vi "DMM Mixed Meas Format Function Range.vi"(0 "DMM Handle In":refnum<k15>, 5 "Function Settings In":T1={"Range and Function"=enum."DC Voltage Auto Range", "Resolution in Digits"=5.5} {"Resolution in Digits" items=["3 1/2"=3.5, "4 1/2"=4.5, "5 1/2"=5.5, "6 1/2"=6.5, "7 1/2"=7.5]}, 11 "error in":errorcluster) -> (4 "DMM Handle Out":refnum<k15>, 6 "Function Settings Out":T4={"Range"=0.0, "Function"=enum."DC Volts", "AC Range"=0.0, "Resolution in Digits"=5.5} {"Resolution in Digits" items=["3 1/2"=3.5, "4 1/2"=4.5, "5 1/2"=5.5, "6 1/2"=6.5, "7 1/2"=7.5]}, 15 "error out":errorcluster)   [LabVIEW 2021, in "DMM_Mixed Measurement.lvlib"]
doc: "Utilizes the function settings input to select the particular function and range used for the measurement and format the output string displayed in the measurement output cluster."
uses:
  DMM_Mixed Measurement.lvlib
  <instrlib>/niDMM/nidmm.llb/niDMM Function.ctl
  <instrlib>/niDMM/nidmm.llb/niDMM Resolution in Digits.ctl
  DMM Mixed Meas Typedefs/Function Settings.ctl
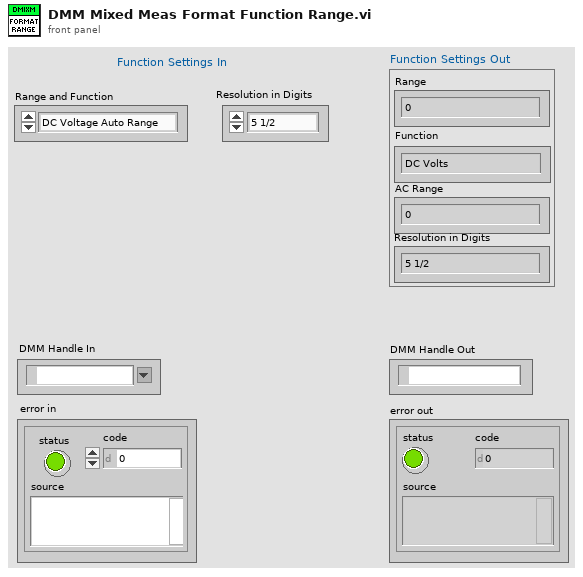
[diagram p1: front panel]
types:
  T1 = typedef "DMM_Mixed Measurement.lvlib/Function Settings.ctl" = cluster{"Range and Function":enum16{"DC Voltage Auto Range", "DC 100 mV", "DC 1 V ", "DC 10 V", "DC 100 V", "DC 300 V", " ", "AC Voltage Auto Range", "AC 50 mV", "AC 200 mV", "AC 500 mV", "AC 2 V", "AC 5 V", "AC 20 V", "AC 50 V", "AC 300 V", "  ", "DC Current Auto Range", "DC 1 uA", "DC 10 uA", "DC 100 uA", "DC 1 mA", "DC 10 mA", "DC 20 mA", "DC 100 mA", "DC 200 mA", "DC 1 A", "DC 3 A", "   ", "AC Current Auto Range", "AC 100 uA", "AC 1 mA", "AC 10 mA", "AC 100 mA", "AC 500 mA", "AC 1 A", "AC 3 A", "    ", "Resistance Auto Range", "Res 100 Ohm", "Res 1 kOhm", "Res 10 kOhm", "Res 100 kOhm", "Res 1 MOhm", "Res 10 MOhm", "Res 100 MOhm", "Res 5 GOhm", "     ", "Frequency AC Auto Range", "Freq AC 50 mV", "Freq AC 500 mV", "Freq AC 5 V", "Freq AC 50 V", "Freq AC 300 V", "      ", "Period AC Auto Range", "Period AC 50 mV", "Period AC 500 mV", "Period AC 5 V", "Period AC 50 V", "Period AC 300 V"}, "Resolution in Digits":T2}
  T2 = typedef "niDMM Resolution in Digits.ctl" = dbl
  T3 = typedef "niDMM Function.ctl" = enum16{"DC Volts", "AC Volts", "DC Current", "AC Current", "2-wire Resistance", "4-wire Resistance", "Diode", "Frequency", "Period", "AC Volts DC Coupled", "Capacitance", "Inductance", "Temperature"}
  T4 = cluster{"Range":dbl, "Function":T3, "AC Range":dbl, "Resolution in Digits":T2}
  T5 = cluster{"Range":dbl, "Function":T3, "Freq_Period AC Range":dbl, "Resolution in Digits":T2}
  T6 = enum16{"DC Voltage Auto Range", "DC 100 mV", "DC 1 V ", "DC 10 V", "DC 100 V", "DC 300 V", " ", "AC Voltage Auto Range", "AC 50 mV", "AC 200 mV", "AC 500 mV", "AC 2 V", "AC 5 V", "AC 20 V", "AC 50 V", "AC 300 V", "  ", "DC Current Auto Range", "DC 1 uA", "DC 10 uA", "DC 100 uA", "DC 1 mA", "DC 10 mA", "DC 20 mA", "DC 100 mA", "DC 200 mA", "DC 1 A", "DC 3 A", "   ", "AC Current Auto Range", "AC 100 uA", "AC 1 mA", "AC 10 mA", "AC 100 mA", "AC 500 mA", "AC 1 A", "AC 3 A", "    ", "Resistance Auto Range", "Res 100 Ohm", "Res 1 kOhm", "Res 10 kOhm", "Res 100 kOhm", "Res 1 MOhm", "Res 10 MOhm", "Res 100 MOhm", "Res 5 GOhm", "     ", "Frequency AC Auto Range", "Freq AC 50 mV", "Freq AC 500 mV", "Freq AC 5 V", "Freq AC 50 V", "Freq AC 300 V", "      ", "Period AC Auto Range", "Period AC 50 mV", "Period AC 500 mV", "Period AC 5 V", "Period AC 50 V", "Period AC 300 V"}
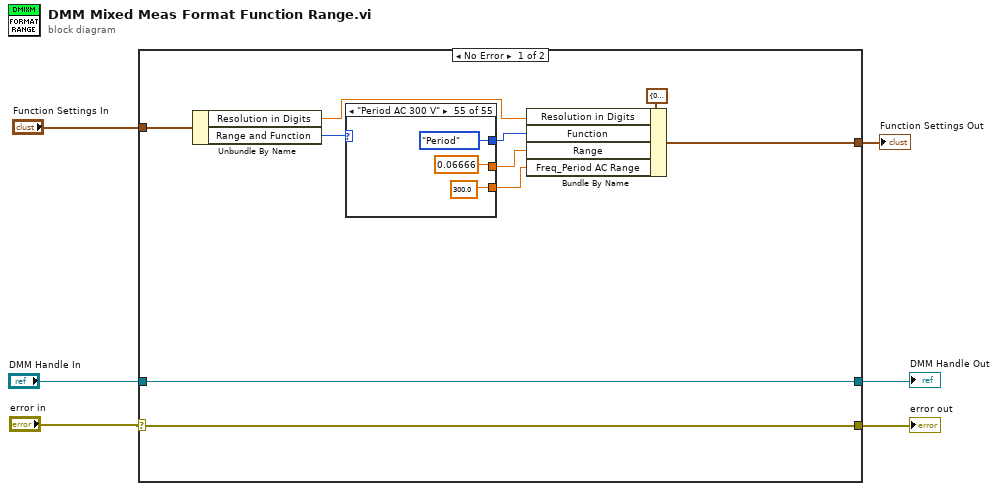
[diagram p0: block diagram]
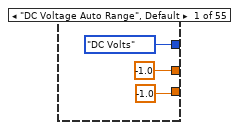
[diagram p2: hidden frame]
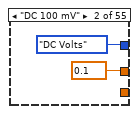
[diagram p3: hidden frame]
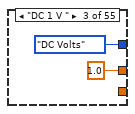
[diagram p4: hidden frame]
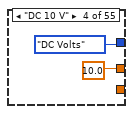
[diagram p5: hidden frame]
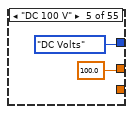
[diagram p6: hidden frame]
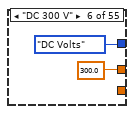
[diagram p7: hidden frame]
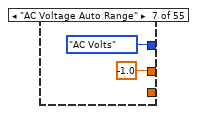
[diagram p8: hidden frame]
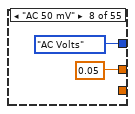
[diagram p9: hidden frame]
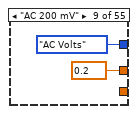
[diagram p10: hidden frame]
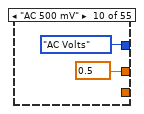
[diagram p11: hidden frame]
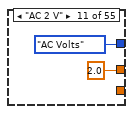
[diagram p12: hidden frame]
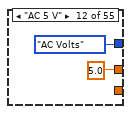
[diagram p13: hidden frame]
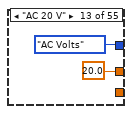
[diagram p14: hidden frame]
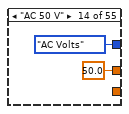
[diagram p15: hidden frame]
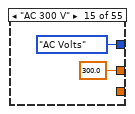
[diagram p16: hidden frame]
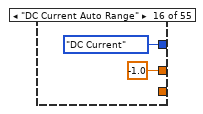
[diagram p17: hidden frame]
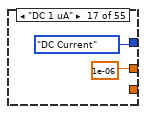
[diagram p18: hidden frame]
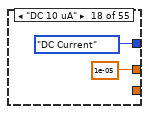
[diagram p19: hidden frame]
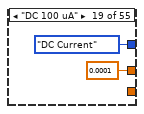
[diagram p20: hidden frame]
diagram:
  n1 = case shown="No Error" "error in" {
    selector: "error in" -> [w8 w141]
    tunnel: "Function Settings In" -> [w16 _]
    tunnel: [w9 T5 {"Range"=-1.0, "Function"=enum."DC Volts", "Freq_Period AC Range"=-1.0, "Resolution in Digits"=5.5} ("Function Settings")] -> w2
    tunnel: [w8 w141] -> w5
    tunnel: [w7 w142] -> w3
    tunnel: "DMM Handle In" -> [w7 w142]
    frame No Error {
      n2 = Unbundle By Name(w16) -> ("Resolution in Digits"=w14:T2, "Range and Function"=w15:T6)
      n3 = case shown="\"Period AC 300 V\"" w15 {
        tunnel: [niDMM_Function."DC Volts" ("Function") niDMM_Function."DC Volts" ("Function") niDMM_Function."DC Volts" ("Function") niDMM_Function."DC Volts" ("Function") niDMM_Function."DC Volts" ("Function") niDMM_Function."DC Volts" ("Function") niDMM_Function."AC Volts" ("Function") niDMM_Function."AC Volts" ("Function") niDMM_Function."AC Volts" ("Function") niDMM_Function."AC Volts" ("Function") niDMM_Function."AC Volts" ("Function") niDMM_Function."AC Volts" ("Function") niDMM_Function."AC Volts" ("Function") niDMM_Function."AC Volts" ("Function") niDMM_Function."AC Volts" ("Function") niDMM_Function."DC Current" ("Function") niDMM_Function."DC Current" ("Function") niDMM_Function."DC Current" ("Function") niDMM_Function."DC Current" ("Function") niDMM_Function."DC Current" ("Function") niDMM_Function."DC Current" ("Function") niDMM_Function."DC Current" ("Function") niDMM_Function."DC Current" ("Function") niDMM_Function."DC Current" ("Function") niDMM_Function."DC Current" ("Function") niDMM_Function."DC Current" ("Function") niDMM_Function."AC Current" ("Function") niDMM_Function."AC Current" ("Function") niDMM_Function."AC Current" ("Function") niDMM_Function."AC Current" ("Function") niDMM_Function."AC Current" ("Function") niDMM_Function."AC Current" ("Function") niDMM_Function."AC Current" ("Function") niDMM_Function."AC Current" ("Function") niDMM_Function."2-wire Resistance" ("Function") niDMM_Function."2-wire Resistance" ("Function") niDMM_Function."2-wire Resistance" ("Function") niDMM_Function."2-wire Resistance" ("Function") niDMM_Function."2-wire Resistance" ("Function") niDMM_Function."2-wire Resistance" ("Function") niDMM_Function."2-wire Resistance" ("Function") niDMM_Function."2-wire Resistance" ("Function") niDMM_Function."2-wire Resistance" ("Function") niDMM_Function."Frequency" ("Function") niDMM_Function."Frequency" ("Function") niDMM_Function."Frequency" ("Function") niDMM_Function."Frequency" ("Function") niDMM_Function."Frequency" ("Function") niDMM_Function."Frequency" ("Function") niDMM_Function."Period" ("Function") niDMM_Function."Period" ("Function") niDMM_Function."Period" ("Function") niDMM_Function."Period" ("Function") niDMM_Function."Period" ("Function") niDMM_Function."Period" ("Function")] -> w10
        tunnel: [-1.0 ("Range") 0.1 ("Range") 1.0 ("Range") 10.0 ("Range") 100.0 ("Range") 300.0 ("Range") -1.0 ("Range") 0.05 ("Range") 0.2 ("Range") 0.5 ("Range") 2.0 ("Range") 5.0 ("Range") 20.0 ("Range") 50.0 ("Range") 300.0 ("Range") -1.0 ("Range") 1e-06 ("Range") 1e-05 ("Range") 0.0001 ("Range") 0.001 ("Range") 0.01 ("Range") 0.02 ("Range") 0.1 ("Range") 0.2 ("Range") 1.0 ("Range") 3.0 ("Range") -1.0 ("Range") 0.0001 ("Range") 0.001 ("Range") 0.01 ("Range") 0.1 ("Range") 0.5 ("Range") 1.0 ("Range") 3.0 ("Range") -1.0 ("Range") 100.0 ("Range") 1000.0 ("Range") 10000.0 ("Range") 100000.0 ("Range") 1000000.0 ("Range") 10000000.0 ("Range") 100000000.0 ("Range") 5000000000.0 ("Range") -1.0 ("Range") 15.0 ("Range") 15.0 ("Range") 15.0 ("Range") 15.0 ("Range") 15.0 ("Range") -1.0 ("Range") 0.06666 ("Range") 0.06666 ("Range") 0.06666 ("Range") 0.06666 ("Range") 0.06666 ("Range")] -> w11
        tunnel: [-1.0 ("Range") _ _ _ _ _ _ _ _ _ _ _ _ _ _ _ _ _ _ _ _ _ _ _ _ _ _ _ _ _ _ _ _ _ _ _ _ _ _ _ _ _ _ -1.0 ("Range") 0.05 ("Range") 0.5 ("Range") 5.0 ("Range") 50.0 ("Range") 300.0 ("Range") -1.0 ("Range") 0.05 ("Range") 0.5 ("Range") 5.0 ("Range") 50.0 ("Range") 300.0 ("Range")] -> w12
        frame "DC Voltage Auto Range", Default {
        }
        frame "DC 100 mV" {
        }
        frame "DC 1 V " {
        }
        frame "DC 10 V" {
        }
        frame "DC 100 V" {
        }
        frame "DC 300 V" {
        }
        frame "AC Voltage Auto Range" {
        }
        frame "AC 50 mV" {
        }
        frame "AC 200 mV" {
        }
        frame "AC 500 mV" {
        }
        frame "AC 2 V" {
        }
        frame "AC 5 V" {
        }
        frame "AC 20 V" {
        }
        frame "AC 50 V" {
        }
        frame "AC 300 V" {
        }
        frame "DC Current Auto Range" {
        }
        frame "DC 1 uA" {
        }
        frame "DC 10 uA" {
        }
        frame "DC 100 uA" {
        }
        frame "DC 1 mA" {
        }
        frame "DC 10 mA" {
        }
        frame "DC 20 mA" {
        }
        frame "DC 100 mA" {
        }
        frame "DC 200 mA" {
        }
        frame "DC 1 A" {
        }
        frame "DC 3 A" {
        }
        frame "AC Current Auto Range" {
        }
        frame "AC 100 uA" {
        }
        frame "AC 1 mA" {
        }
        frame "AC 10 mA" {
        }
        frame "AC 100 mA" {
        }
        frame "AC 500 mA" {
        }
        frame "AC 1 A" {
        }
        frame "AC 3 A" {
        }
        frame "Resistance Auto Range" {
        }
        frame "Res 100 Ohm" {
        }
        frame "Res 1 kOhm" {
        }
        frame "Res 10 kOhm" {
        }
        frame "Res 100 kOhm" {
        }
        frame "Res 1 MOhm" {
        }
        frame "Res 10 MOhm" {
        }
        frame "Res 100 MOhm" {
        }
        frame "Res 5 GOhm" {
        }
        frame "Frequency AC Auto Range" {
          # "Amplitude"
          # "Hz"
        }
        frame "Freq AC 50 mV" {
        }
        frame "Freq AC 500 mV" {
        }
        frame "Freq AC 5 V" {
        }
        frame "Freq AC 50 V" {
        }
        frame "Freq AC 300 V" {
        }
        frame "Period AC Auto Range" {
          # "Amplitude"
          # "s"
        }
        frame "Period AC 50 mV" {
        }
        frame "Period AC 500 mV" {
        }
        frame "Period AC 5 V" {
        }
        frame "Period AC 50 V" {
        }
        frame "Period AC 300 V" {
        }
      }
      n4 = Bundle By Name(cluster=T5 {"Range"=0.1, "Function"=enum."DC Volts", "Freq_Period AC Range"=0.1, "Resolution in Digits"=5.5} ("Function Settings"), "Resolution in Digits"=w14, "Function"=w10, "Range"=w11, "Freq_Period AC Range"=w12) -> (w9:T5)
    }
    frame Error {
    }
  }
  "error out" <- w5
  "DMM Handle Out" <- w3
  "Function Settings Out" <- w2
